vi "Request Compatible Hardware.vi"(8 "error in (no error)":errorcluster, 11 "Msmt UI in":refnum<class "Measurement UI.lvclass">) -> (0 "error out":errorcluster, 3 "Msmt UI out":refnum<class "Measurement UI.lvclass">)   [LabVIEW 2016, in "Measurement UI.lvlib" / "Measurement UI.lvclass"]
uses:
  Measurement UI.lvclass
  C:/Program Files (x86)/National Instruments/LabVIEW 2016/vi.lib/ActorFramework/Actor/Actor.lvclass
  Measurement UI.lvclass/Measurement UI.ctl
  <vilib>/ActorFramework/Actor/Actor.lvclass/Actor.ctl
  Controller/Messages/Find Compatible Hardware for Measurement Msg/Find Compatible Hardware for Measurement Msg.lvclass/Find Compatible Hardware for Measurement Msg.ctl
  <vilib>/ActorFramework/Message Enqueuer/Message Enqueuer.lvclass/Message Enqueuer.ctl
  Accessors/Read Measurement.vi
  <vilib>/ActorFramework/Message Enqueuer/Enqueue.vi
  Controller/Messages/Find Compatible Hardware for Measurement Msg/Find Compatible Hardware for Measurement Msg.lvclass
  C:/Program Files (x86)/National Instruments/LabVIEW 2016/vi.lib/ActorFramework/Message/Message.lvclass
  <vilib>/ActorFramework/Message Priority Queue/Priority Enqueue.vi
  <vilib>/ActorFramework/Actor/Actor.lvclass
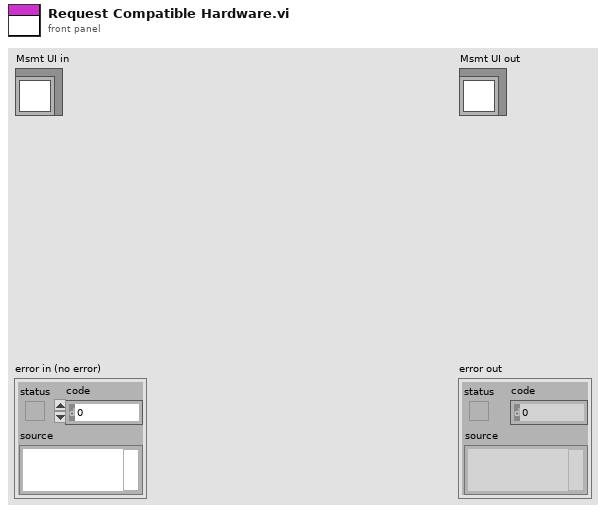
[diagram p1: front panel]
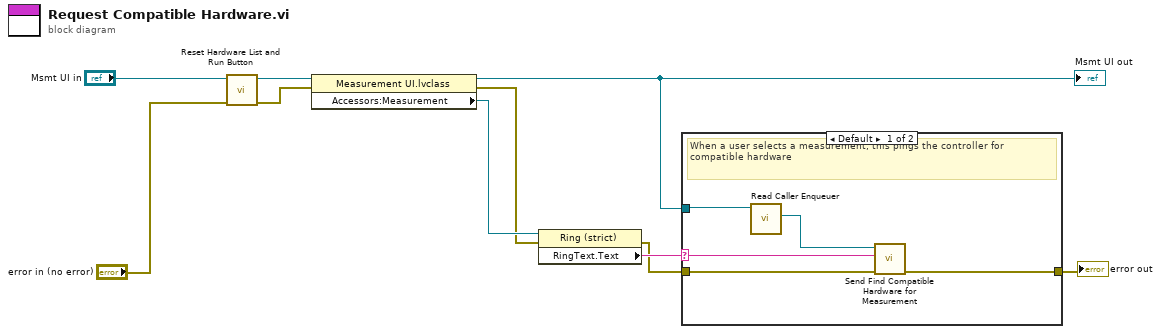
[diagram p0: block diagram]
diagram:
  n1 = call "Reset Hardware List and Run Button.vi"("error in (no error)"="error in (no error)", "Measurement UI in"="Msmt UI in") -> ("error out"=w2:errorcluster, "Measurement UI out"=w8:refnum<class "Measurement UI.lvclass">)  [unwired: 8 in]
  n2 = property class="Measurement UI.lvclass"(reference=w8, error in=w2) -> (reference out=w7:refnum<class "Measurement UI.lvclass">, error out=w4:errorcluster, "Accessors:Measurement"=w6:refnum<vi>)
  "Msmt UI out" <- w7
  n3 = property class="Ring (strict)"(reference=w6, error in=w4) -> (error out=w3:errorcluster, "RingText.Text"=w10:string)  [unwired: 1 out]
  n4 = case shown="Default" w10 {
    selector: w10 -> [w13 _]
    tunnel: w7 -> [w15 _]
    tunnel: w3 -> [w12 w16]
    tunnel: [w11 w16] -> w1
    frame Default {
      # "When a user selects a measurement, this pings the controller for compatible hardware"
      n5 = call <vilib>:"Read Caller Enqueuer.vi"("Actor"=w15) -> ("Caller Enqueuer"=w14:refnum<class "Message Enqueuer.lvclass">)  [unwired: 10 in]
      n6 = call "Send Find Compatible Hardware for Measurement.vi"("error in (no error)"=w12, "Measurement Name"=w13, "Message Enqueuer"=w14) -> ("error out"=w11:errorcluster)  [unwired: 7 in, 1 out]
    }
    frame "Select One:" {
    }
  }
  "error out" <- w1
